vi "SensorASCIIProcessor.vi"(6 "Notifier Error In":errorcluster, 7 "Shutdown Notifier":refnum<notifier>, 8 "Queue":refnum<queue>) -> (1 "Notifier Error Out":errorcluster, 3 "Done":bool)   [LabVIEW 2013]
uses:
  SensorDataType.ctl
panel:
  out "Sensor Data (normalized)":dbl[](array[numeric])
  out "Sensor Line Buffer":string
  out "Sensor Data (raw)":dbl[](array[numeric])
  out "current sensor line ASCII":string
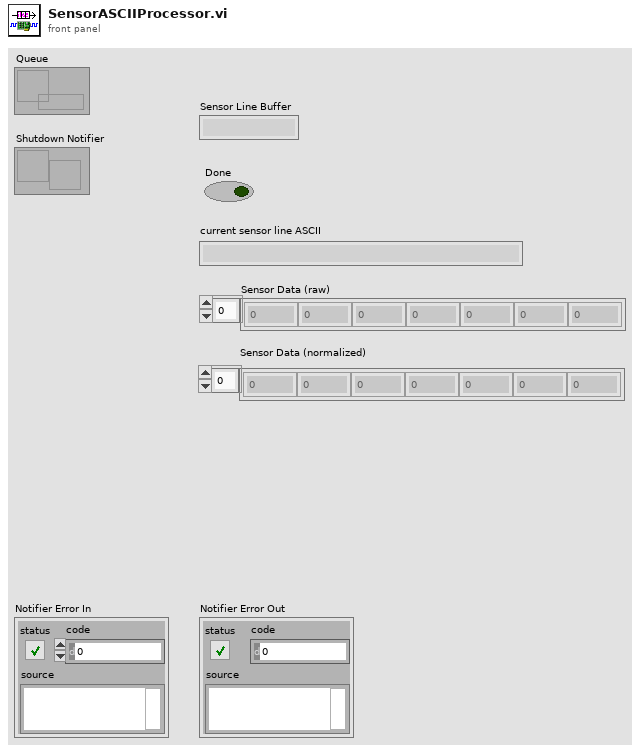
[diagram p1: front panel]
types:
  T1 = typedef "SensorDataType.ctl" = cluster{"Raw":u16[], "Normalized\n":dbl[]}
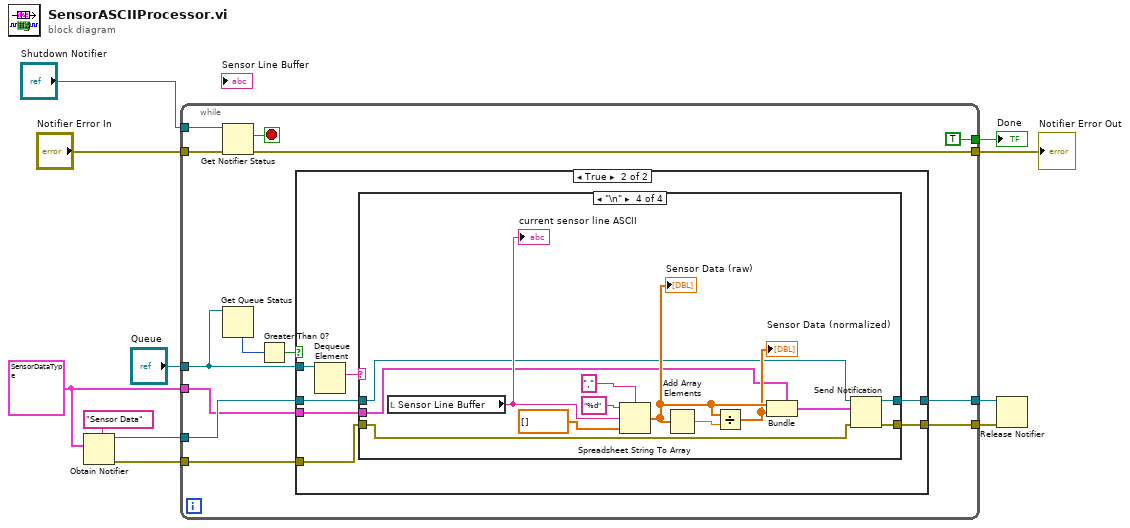
[diagram p0: block diagram]
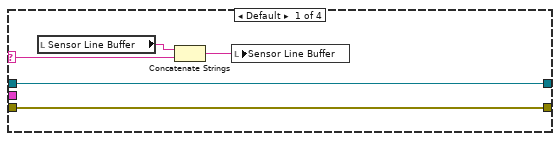
[diagram p3: hidden frame]
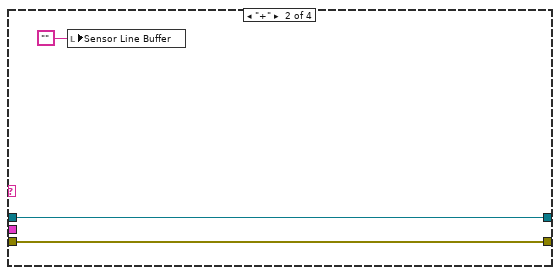
[diagram p4: hidden frame]
diagram:
  w4 = T1 {"Raw"=[22, 22, 26, 24, 24, 26, 26], "Normalized\n"=[0.12941176470588237, 0.12941176470588237, 0.15294117647058825, 0.1411764705882353, 0.1411764705882353, 0.15294117647058825, 0.15294117647058825]} ("Sensor Data Type")
  n1 = Obtain Notifier(name (unnamed)="Sensor Data", notification data type=w4) -> (notifier out=w6:refnum<notifier>, error out=w1:errorcluster)  [unwired: 2 in, 1 out]
  n2 = while {
    tunnel: "Queue" -> [w19]
    tunnel: "Shutdown Notifier" -> [w23]
    tunnel: [w21] -> w7
    tunnel: "Notifier Error In" -> [w20]
    tunnel: [TRUE] -> w11
    tunnel: w6 -> [w16]
    tunnel: w4 -> [w15]
    tunnel: [w14] -> w3
    tunnel: [w13] -> w2
    tunnel: w1 -> [w12]
    stop <- w22 stop-if-true
    n3 = Get Notifier Status(notifier=w23, error in (no error)=w20) -> (current notification=w22:bool, error out=w21:errorcluster)  [unwired: 3 out]
    n4 = Get Queue Status(queue=w19) -> (# elements in queue=w17:i32)  [unwired: 2 in, 7 out]
    n5 = Greater Than 0?(x=w17) -> (x > 0?=w24:bool)
    n6 = case shown="True" w24 {
      tunnel: w19 -> [_ w33]
      tunnel: w16 -> [w25 w31]
      tunnel: w15 -> [_ w30]
      tunnel: [w25 w29] -> w14
      tunnel: [w26 w28] -> w13
      tunnel: w12 -> [w26 w27]
      frame False {
      }
      frame True {
        n7 = Dequeue Element(queue=w33) -> (element=w32:string)  [unwired: 2 in, 3 out]
        n8 = case shown="\"\\n\"" w32 {
          selector: w32 -> [w38 _ _ _]
          tunnel: w31 -> [w34 w39 w42 w48]
          tunnel: w30 -> [_ _ _ w47]
          tunnel: [w34 w39 w42 w46] -> w29
          tunnel: [w35 w40 w43 w45] -> w28
          tunnel: w27 -> [w35 w40 w43 w44]
          frame Default {
            n9 = local read "Sensor Line Buffer"() -> (w36:string)
            n10 = Concatenate Strings(w36, w38) -> (w37:string)
            n11 = local write "Sensor Line Buffer"(w37) -> ()
          }
          frame "+" {
            n12 = local write "Sensor Line Buffer"("") -> ()
          }
          frame "\r" {
          }
          frame "\n" {
            n13 = local read "Sensor Line Buffer"() -> (w52:string)
            "current sensor line ASCII" <- w52
            n14 = Spreadsheet String To Array(delimiter (Tab)=",", format string="%d", spreadsheet string=w52, array type (2D Dbl)=dbl[] []) -> (array=w51:dbl[])
            "Sensor Data (raw)" <- w51
            n15 = Add Array Elements(numeric array=w51) -> (sum=w53:dbl)
            n16 = Divide(x=w51, y=w53) -> (x/y=w50:dbl[])
            "Sensor Data (normalized)" <- w50
            n17 = Bundle(cluster=w47, "Raw"=w51, "Normalized"=w50) -> (w49:T1)
            n18 = Send Notification(notification=w49, notifier=w48, error in (no error)=w44) -> (notifier out=w46:refnum<notifier>, error out=w45:errorcluster)
          }
        }
      }
    }
  }
  "Done" <- w11
  "Notifier Error Out" <- w7
  n19 = Release Notifier(notifier=w3, error in (no error)=w2) -> ()  [unwired: 1 in, 3 out]
